vi "命令模式DEMO(简单）.vi"() -> ()   [LabVIEW 2013]
uses:
  Panel_class/Panel.lvclass
  Command_class/Command.lvclass
  Spindle_class/Spindle.lvclass
  SpindleOnCommand_class/SpindleOnCommand.lvclass
  <vilib>/addons/_AddQ/G#Object/G#Object.lvclass
  SpindleOffCommand_class/SpindleOffCommand.lvclass
panel:
  in  "Y Axis":bool
  in  "停止":bool
  in  "X Axis":bool
  out "# of objects killed 2":i32
  out "Output":string
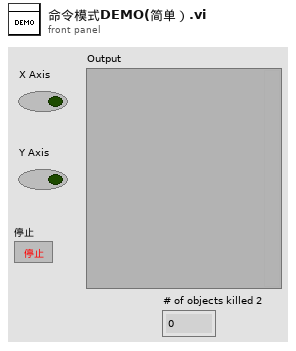
[diagram p1: front panel]
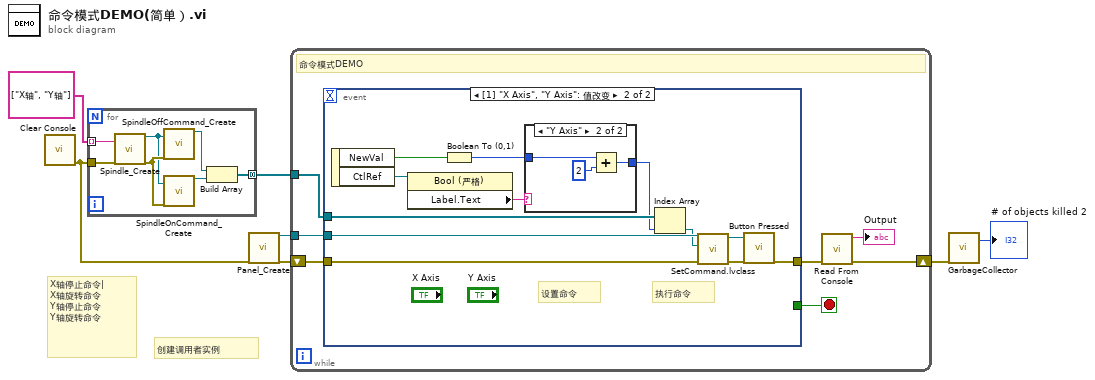
[diagram p0: block diagram]
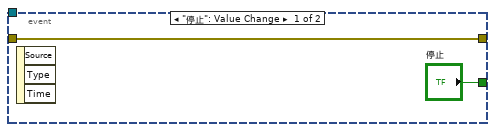
[diagram p2: hidden frame]
diagram:
  # "创建调用者实例"
  # "X轴停止命令|\nX轴旋转命令\nY轴停止命令\nY轴旋转命令"
  n1 = call "Clear Console.vi"() -> ("error out"=w1:errorcluster)  [unwired: 11 in]
  n2 = for {
    tunnel: string[] ["X轴", "Y轴"] -> [w14] mode=indexing
    tunnel: [w9] -> w2 mode=concatenating
    tunnel: w1 -> [w8]
    n3 = call "Spindle_Create.vi"("Name"=w14, "error in (no error)"=w8) -> ("reference out"=w12:refnum<class "Spindle.lvclass">, "error out"=w13:errorcluster)  [unwired: 16 in]
    n4 = call "SpindleOffCommand_Create.vi"("Spindle.lvclass"=w12, "error in (no error)"=w13) -> ("reference out"=w11:refnum<class "SpindleOffCommand.lvclass">)  [unwired: 16 in, 1 out]
    n5 = call "SpindleOnCommand_Create.vi"("Spindle.lvclass"=w12, "error in (no error)"=w13) -> ("reference out"=w10:refnum<class "SpindleOnCommand.lvclass">)  [unwired: 16 in, 1 out]
    n6 = Build Array(w11, w10) -> (w9:refnum<class "Command.lvclass">[])
  }
  n7 = call "Panel_Create.vi"("error in (no error)"=w1) -> ("reference out"=w6:refnum<class "Panel.lvclass">, "error out"=w5:errorcluster)  [unwired: 17 in]
  n8 = while {
    tunnel: w6 -> [w19]
    shift-right: [w17] -> w4
    shift-left: w5 -> [w20]
    tunnel: w2 -> [w15]
    stop <- w21 stop-if-true
    # "命令模式DEMO"
    n9 = event shown="[1] \"X Axis\", \"Y Axis\": 值改变" {
      selector: _ -> [_ _]
      dyn-events: _ -> [_ _]
      timeout: _ -> [_ _]
      tunnel: ["停止" _] -> w21
      tunnel: w20 -> [w22 w33]
      tunnel: [w22 w35] -> w18
      tunnel: w19 -> [_ w34]
      tunnel: w15 -> [_ w30]
      event "停止": Value Change {
        n10 = event-data() -> ()  [unwired: 1 in, 3 out]
      }
      event "X Axis", "Y Axis": Value Change {
        # "执行命令"
        # "设置命令"
        n11 = event-data() -> ("NewVal"=w26:bool, "CtlRef"=w28:refnum<vi>)  [unwired: 1 in]
        n12 = property class="Bool (严格)"(reference=w28) -> ("Label.Text"=w27:string)  [unwired: 1 in, 2 out]
        n13 = Boolean To (0,1)(Boolean=w26) -> (0, 1=w25:i16)
        n14 = case shown="\"Y Axis\"" w27 {
          tunnel: w25 -> [w36 w39]
          tunnel: [w36 w37] -> w24
          frame "X Axis", Default {
          }
          frame "Y Axis" {
            n15 = Add(x=w39, y=i16 2) -> (x+y=w37:i16)
          }
        }
        n16 = Index Array(array=w30, index=w24) -> (element=w29:refnum<class "Command.lvclass">)
        n17 = call-dynamic "SetCommand.lvclass.vi"("error in (no error)"=w33, "Command.lvclass"=w29, "reference in"=w34) -> ("error out"=w32:errorcluster, "reference out"=w31:refnum<class "Panel.lvclass">)  [unwired: 7 in]
        n18 = call-dynamic "Button Pressed.vi"("reference in"=w31, "error in (no error)"=w32) -> ("error out"=w35:errorcluster)  [unwired: 16 in, 1 out]
      }
    }
    n19 = call "Read From Console.vi"("error in (no error)"=w18) -> ("error out"=w17:errorcluster, "Output"=→"Output":string)  [unwired: 9 in]
  }
  n20 = call <vilib>:"GarbageCollector.vi"("error in (no error)"=w4) -> ("# of objects killed"=→"# of objects killed 2":i32)  [unwired: 16 in, 2 out]
